vi "Parse Formula String.vi"(2 "error in (no error)":errorcluster, 3 "formula":string) -> (0 "error out":errorcluster, 1 "Parsed Formula":cluster{"Table":i32[][], "Y Values":dbl[]} {"Y Values" format="%.2f"})   [LabVIEW 2020, in "NI_Gmath.lvlib"]
doc: "Analyzes a string as a formula and produces two numeric arrays. These arrays can be used by the Eval Parsed Formula String VI."
uses:
  <vilib>/gmath/NI_Gmath.lvlib
panel:
  # "Example:\n\n formula: x*sinh(z)+7*y"
  # "operator"
  # "register1"
  # "register2"
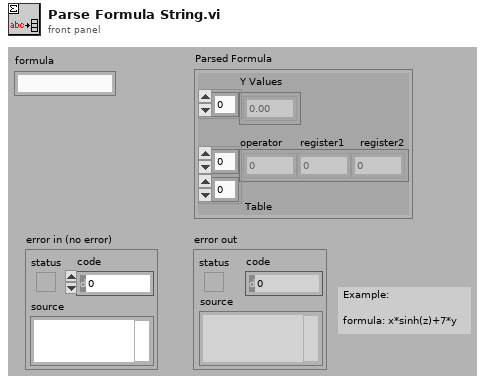
[diagram p1: front panel]
types:
  T1 = cluster{"text":string, "left":i32, "right":i32, "father":i32}[]
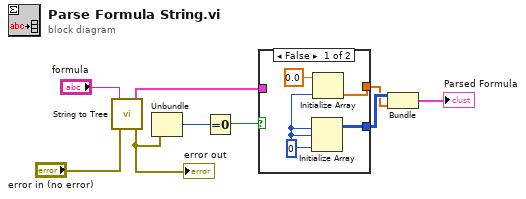
[diagram p0: block diagram]
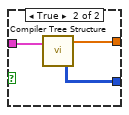
[diagram p2: hidden frame]
diagram:
  n1 = call <vilib>:"String to Tree.VI"("error in (no error)"="error in (no error)", "user formula"="formula") -> ("error out"=w1:errorcluster, "Tree formula"=w8:T1)
  "error out" <- w1
  n2 = Unbundle(w1) -> ("code"=w6:i32)  [unwired: 2 out]
  n3 = Equal To 0?(x=w6) -> (x = 0?=w9:bool)
  n4 = case shown="False" w9 {
    tunnel: w8 -> [_ w16]
    tunnel: [w11 w15] -> w4
    tunnel: [w10 w14] -> w5
    frame False {
      w13 = 0
      n5 = Initialize Array(w13, w13, w13) -> (w10:i32[][])
      n6 = Initialize Array(0.0, w13) -> (w11:dbl[])
    }
    frame True {
      n7 = call <vilib>:"Compiler Tree Structure.VI"("Tree formula"=w16) -> ("Result"=w15:dbl[], "Table"=w14:i32[][])
    }
  }
  n8 = Bundle("Table"=w5, "Result"=w4) -> (→"Parsed Formula":cluster{"Table":i32[][], "Result":dbl[]})  [unwired: 1 in]
